vi "testGetSpecificTopic.vi"(8 "error in (no error)":errorcluster) -> (0 "error out":errorcluster)   [LabVIEW 2018]
uses:
  SALTypeGenerator/Module/Module.lvclass
  SALTypeGenerator/Topic/Topic.lvclass
  SALTypeGenerator/Topic/Topic.lvclass/Topic.ctl
  SALTypeGenerator/Module/Module.lvclass/Module.ctl
  <vilib>/addons/_JKI Toolkits/Caraya/classes/Assert/Assert Equal Value_Variant.vi
  <vilib>/addons/_JKI Toolkits/Caraya/classes/Test/Test.lvclass
  <vilib>/addons/_JKI Toolkits/Caraya/classes/Assert/Assert.lvclass
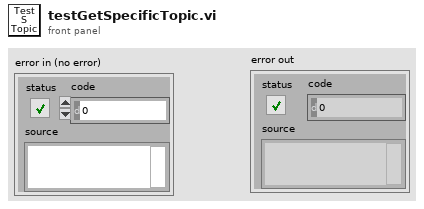
[diagram p1: front panel]
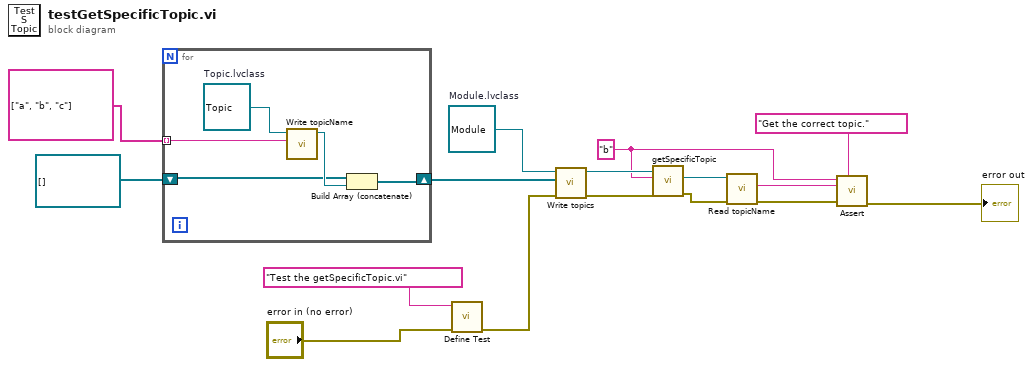
[diagram p0: block diagram]
diagram:
  w3 = "b" ("nameTopic")
  w14 = refnum<class "Module.lvclass"> refnum  # Module.lvclass
  n1 = for {
    tunnel: string[] ["a", "b", "c"] -> [w20] mode=indexing
    shift-right: [w18] -> w13
    shift-left: refnum<class "Topic.lvclass">[] [] -> [w17]
    w21 = refnum<class "Topic.lvclass"> refnum  # Topic.lvclass
    n2 = call "Write topicName.vi"("topicName"=w20, "Topic in"=w21) -> ("Topic out"=w19:refnum<class "Topic.lvclass">)  [unwired: 9 in]
    n3 = Build Array (concatenate)(w17, w19) -> (w18:refnum<class "Topic.lvclass">[])
  }
  n4 = call <vilib>:"Define Test.vi"("error in (no error)"="error in (no error)", "Label (VI Title)"="Test the getSpecificTopic.vi") -> ("error out"=w10:errorcluster)  [unwired: 9 in]
  n5 = call "Write topics.vi"("error in (no error)"=w10, "topics"=w13, "Module in"=w14) -> ("error out"=w8:errorcluster, "Module out"=w9:refnum<class "Module.lvclass">)  [unwired: 7 in]
  n6 = call "getSpecificTopic.vi"("error in (no error)"=w8, "nameTopic"=w3, "Module in"=w9) -> ("error out"=w6:errorcluster, "Topic.lvclass"=w7:refnum<class "Topic.lvclass">)  [unwired: 6 in, 1 out]
  n7 = call "Read topicName.vi"("error in (no error)"=w6, "Topic in"=w7) -> ("error out"=w5:errorcluster, "topicName"=w4:string)  [unwired: 7 in, 1 out]
  n8 = call-poly <vilib>:"Assert.vi"("Label"="Get the correct topic.", "error in (no error)"=w5, "Y"=w4, "X"=w3) -> ("error out"=→"error out":errorcluster)  [unwired: 7 in]
